vi "Graph_cursors_minmaxSD.vi"(1 "Max Y pixel":i32, 2 "Max X pixel":i32, 3 "GRAPH EXPERIMENTAL DATA":refnum<vi>) -> (0 "max/min XY pixels":T1)   [LabVIEW 2015]
panel:
  out "Boolean":bool
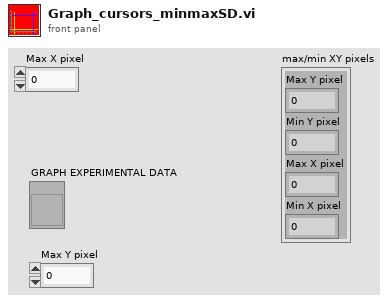
[diagram p1: front panel]
types:
  T1 = cluster{"Max Y pixel":i32, "Min Y pixel":i32, "Max X pixel":i32, "Min X pixel":i32}
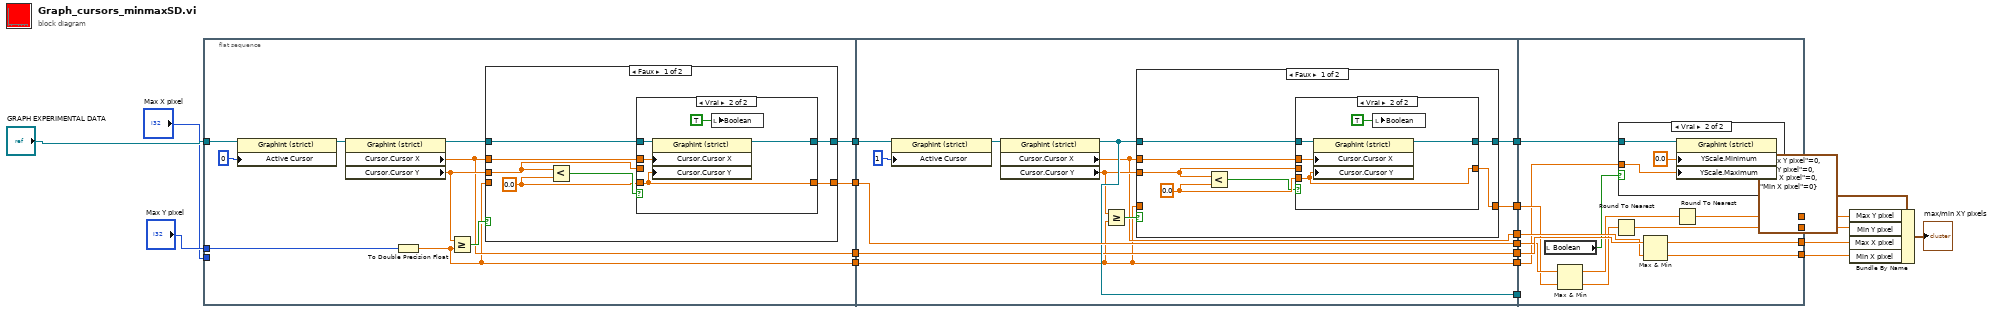
[diagram p0: block diagram]
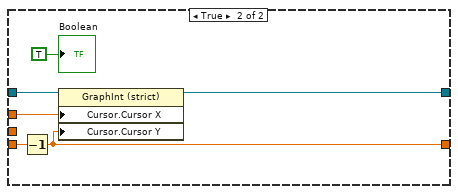
[diagram p3: hidden frame]
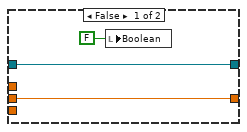
[diagram p4: hidden frame]
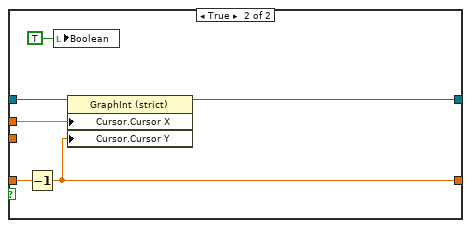
[diagram p5: hidden frame]
diagram:
  n1 = flat-sequence {
    tunnel: [w22] -> w20
    tunnel: "GRAPH EXPERIMENTAL DATA" -> [w30]
    tunnel: [w23] -> w19
    tunnel: [w27] -> w18
    tunnel: "Max Y pixel" -> [w25]
    tunnel: [w21] -> w17
    tunnel: "Max X pixel" -> [_]
    tunnel: w20 -> [w53]
    tunnel: w19 -> [w62]
    tunnel: w18 -> [w61]
    tunnel: [w53] -> w16
    tunnel: [w55] -> w15
    tunnel: [w57] -> w14
    tunnel: [w61] -> w13
    tunnel: [w59] -> w12
    tunnel: w17 -> [w52]
    tunnel: [w54] -> w11
    tunnel: [w52] -> w10
    tunnel: w16 -> [w95]
    tunnel: w15 -> [w94]
    tunnel: w14 -> [w90]
    tunnel: w13 -> [w91]
    tunnel: w12 -> [_]
    tunnel: [w97] -> w2
    tunnel: [w96] -> w1
    tunnel: [w88] -> w6
    tunnel: [w89] -> w5
    tunnel: w11 -> [w87]
    tunnel: w10 -> [w86]
    frame #0 {
      n2 = property on="Property Node" class="GraphInt (strict)"(reference=w30, "Active Cursor"=u32 0) -> (reference out=w29:refnum<vi>)  [unwired: 1 in, 1 out]
      n3 = property on="Property Node" class="GraphInt (strict)"(reference=w29) -> (reference out=w24:refnum<vi>, "Cursor.Cursor X"=w22:dbl, "Cursor.Cursor Y"=w26:dbl)  [unwired: 1 in, 1 out]
      n4 = To Double Precision Float(number=w25) -> (double precision float=w21:dbl)
      n5 = Greater Or Equal?(x=w26, y=w21) -> (x >= y?=w28:bool)
      n6 = case shown="Faux" w28 {
        tunnel: [w37 w49] -> w27
        tunnel: w26 -> [w36 _]
        tunnel: w21 -> [_ w51]
        tunnel: [w34 w48] -> w23
        tunnel: w24 -> [w35 w47]
        tunnel: w22 -> [w32 w50]
        frame False {
          w33 = 0.0 ("y")
          n7 = Less?(x=w36, y=w33) -> (x < y?=w38:bool)
          n8 = case shown="Vrai" w38 {
            tunnel: [w40 w42] -> w37
            tunnel: w36 -> [w40 _]
            tunnel: w35 -> [w39 w45]
            tunnel: [w39 w44] -> w34
            tunnel: w33 -> [_ w42]
            tunnel: w32 -> [_ w43]
            frame False {
            }
            frame True {
              n9 = property on="Property Node" class="GraphInt (strict)"(reference=w45, "Cursor.Cursor X"=w43, "Cursor.Cursor Y"=w42) -> (reference out=w44:refnum<vi>)  [unwired: 1 in, 1 out]
              n10 = local write "Boolean"(TRUE ("Boolean")) -> ()
            }
          }
        }
        frame True {
          n11 = Decrement(x=w51) -> (x-1=w49:dbl)
          n12 = property on="Property Node" class="GraphInt (strict)"(reference=w47, "Cursor.Cursor X"=w50, "Cursor.Cursor Y"=w49) -> (reference out=w48:refnum<vi>)  [unwired: 1 in, 1 out]
          "Boolean" <- TRUE ("Boolean")
        }
      }
    }
    frame #1 {
      n13 = property on="Property Node" class="GraphInt (strict)"(reference=w62, "Active Cursor"=u32 1) -> (reference out=w60:refnum<vi>)  [unwired: 1 in, 1 out]
      n14 = property on="Property Node" class="GraphInt (strict)"(reference=w60) -> (reference out=w59:refnum<vi>, "Cursor.Cursor X"=w55:dbl, "Cursor.Cursor Y"=w56:dbl)  [unwired: 1 in, 1 out]
      n15 = Greater Or Equal?(x=w56, y=w52) -> (x >= y?=w58:bool)
      n16 = case shown="Faux" w58 {
        tunnel: [w64 w82] -> w57
        tunnel: w52 -> [_ w84]
        tunnel: [w66 w81] -> w54
        tunnel: w59 -> [w67 w80]
        tunnel: w55 -> [w65 w83]
        tunnel: w56 -> [w68 _]
        frame False {
          w70 = 0.0 ("y")
          n17 = Less?(x=w68, y=w70) -> (x < y?=w69:bool)
          n18 = case shown="Vrai" w69 {
            tunnel: [w73 w75] -> w64
            tunnel: w68 -> [w73 _]
            tunnel: w67 -> [w72 w78]
            tunnel: [w72 w77] -> w66
            tunnel: w70 -> [_ w75]
            tunnel: w65 -> [_ w76]
            frame False {
              n19 = local write "Boolean"(FALSE ("Boolean")) -> ()
            }
            frame True {
              n20 = property on="Property Node" class="GraphInt (strict)"(reference=w78, "Cursor.Cursor X"=w76, "Cursor.Cursor Y"=w75) -> (reference out=w77:refnum<vi>)  [unwired: 1 in, 1 out]
              n21 = local write "Boolean"(TRUE ("Boolean")) -> ()
            }
          }
        }
        frame True {
          n22 = Decrement(x=w84) -> (x-1=w82:dbl)
          n23 = local write "Boolean"(TRUE ("Boolean")) -> ()
          n24 = property on="Property Node" class="GraphInt (strict)"(reference=w80, "Cursor.Cursor X"=w83, "Cursor.Cursor Y"=w82) -> (reference out=w81:refnum<vi>)  [unwired: 1 in, 1 out]
        }
      }
    }
    frame #2 {
      n25 = local read "Boolean"() -> (w85:bool)
      n26 = Max & Min(x=w91, y=w90) -> (max(x,y)=w93:dbl, min(x,y)=w92:dbl)
      n27 = Round To Nearest(number=w92) -> (nearest integer value=w89:dbl)
      n28 = case shown="Vrai" w85 {
        tunnel: w87 -> [_ w100]
        tunnel: w86 -> [_ w98]
        frame False {
        }
        frame True {
          n29 = property on="Property Node" class="GraphInt (strict)"(reference=w100, "YScale.Minimum"=0.0 ("Y Scale.Range:Minimum"), "YScale.Maximum"=w98) -> ()  [unwired: 1 in, 2 out]
        }
      }
      n30 = Max & Min(x=w95, y=w94) -> (max(x,y)=w97:dbl, min(x,y)=w96:dbl)
      n31 = Round To Nearest(number=w93) -> (nearest integer value=w88:dbl)
    }
  }
  n32 = Bundle By Name(cluster=T1 {"Max Y pixel"=0, "Min Y pixel"=0, "Max X pixel"=0, "Min X pixel"=0}, "Max Y pixel"=w6, "Min Y pixel"=w5, "Max X pixel"=w2, "Min X pixel"=w1) -> (→"max/min XY pixels":T1)
